vi "FPGA SPI_Configure.vi"(8 "error in":errorcluster, 9 "Configuration Cluster":T2={"CS"=1, "Clock Rate (Hz)"=50000.0, "Clock Mode"=0, "CS Active State"=FALSE} {"CS" items=["0"=1, "1"=2, "2"=4, "3"=8, "4"=16, "5"=32, "6"=64, "7"=128]; "Clock Mode" items=["0", "1", "2", "3"]}, 10 "Port":u8, 11 "FPGA VI Reference":T1) -> (0 "error out":errorcluster, 2 "Actual Rate (Hz)":dbl, 3 "FPGA VI Reference Out":T1)   [LabVIEW 2011]
uses:
  <vilib>/rvi/interface/nirviReadWriteControl/nirviReadWriteControl.xnode
  FPGA/Controls/FPGA SPI_Cmd.ctl
  Controls/FPGA SPI_FPGA Ref.ctl
  Controls/FPGA SPI_SPI Configuration Cluster.ctl
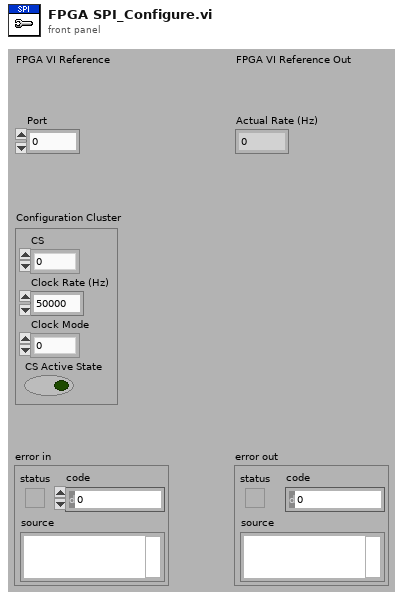
[diagram p1: front panel]
types:
  T1 = typedef "FPGA SPI_FPGA Ref.ctl" = refnum<k20>
  T2 = typedef "FPGA SPI_SPI Configuration Cluster.ctl" = cluster{"CS":u8, "Clock Rate (Hz)":dbl, "Clock Mode":u8, "CS Active State":bool}
  T3 = typedef "FPGA SPI_Cmd.ctl" = enum8{"Idle", "Write/Read SPI", "Configure"}
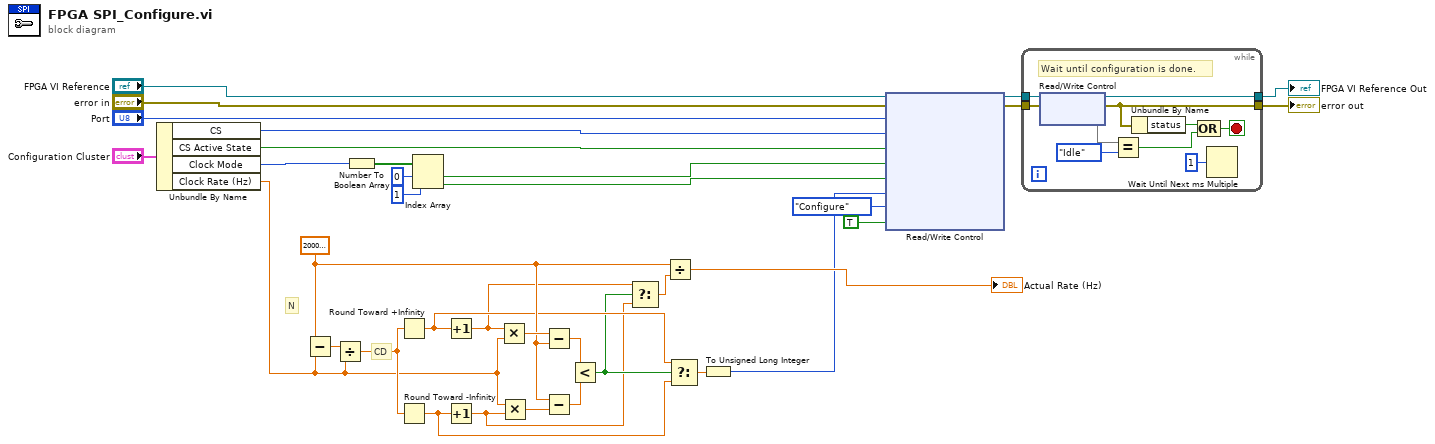
[diagram p0: block diagram]
diagram:
  w26 = 20000000.0 ("10M")
  # "CD"
  # "N"
  n1 = Unbundle By Name("Configuration Cluster") -> ("CS"=w31:u8, "CS Active State"=w8:bool, "Clock Mode"=w9:u8, "Clock Rate (Hz)"=w15:dbl)
  n2 = Subtract(x=w26, y=w15) -> (x-y=w25:dbl)
  n3 = Divide(x=w25, y=w15) -> (x/y=w24:dbl)
  n4 = Number To Boolean Array(number=w9) -> (Boolean array=w14:bool[])
  n5 = Round Toward +Infinity(x=w24) -> (ceil(x): smallest int >= x=w23:dbl)
  n6 = Round Toward -Infinity(1:w24) -> (0:w22:dbl)
  n7 = Index Array(array=w14, index #1=0 ("index"), index #2=1 ("index")) -> (element #1=w11:bool, element #2=w10:bool)
  n8 = Increment(x=w23) -> (x+1=w18:dbl)
  n9 = Increment(x=w22) -> (x+1=w19:dbl)
  n10 = Multiply(x=w18, y=w15) -> (x*y=w30:dbl)
  n11 = Multiply(x=w15, y=w19) -> (x*y=w29:dbl)
  n12 = Subtract(x=w30, y=w26) -> (x-y=w27:dbl)
  n13 = Subtract(x=w26, y=w29) -> (x-y=w28:dbl)
  n14 = Less?(x=w27, y=w28) -> (x < y?=w20:bool)
  n15 = Select(t=w18, s=w20, f=w19) -> (s? t:f=w21:dbl)
  n16 = Divide(x=w26, y=w21) -> (x/y=→"Actual Rate (Hz)":dbl)
  n17 = Select(t=w23, s=w20, f=w22) -> (s? t:f=w16:dbl)
  n18 = To Unsigned Long Integer(number=w16) -> (unsigned 32bit integer=w7:u32)
  n19 = xnode "Read/Write Control"("FPGA VI Reference In"="FPGA VI Reference", "error in"="error in", "SPI_Port"="Port", "SPI_CS"=w31, "SPI_CS Active State"=w8, "SPI_CPHA"=w11, "SPI_CPOL"=w10, "SPI_Clock Divider"=w7, "SPI_Cmd"=FPGA_SPI_Cmd."Configure" ("Cmd"), "SPI_Start"=TRUE ("Start")) -> ("FPGA VI Reference Out"=w4:T1, "error out"=w2:errorcluster)
  n20 = while {
    tunnel: w4 -> [w45]
    tunnel: [w44] -> w3
    tunnel: w2 -> [w43]
    tunnel: [w40] -> w1
    stop <- w37 stop-if-true
    # "Wait until configuration is done."
    n21 = xnode "Read/Write Control"("FPGA VI Reference In"=w45, "error in"=w43) -> ("FPGA VI Reference Out"=w44:T1, "error out"=w40:errorcluster, "SPI_Cmd"=w42)
    n22 = Equal?(x=w42, y=FPGA_SPI_Cmd."Idle") -> (x = y?=w38:bool)
    n23 = Unbundle By Name(w40) -> ("status"=w39:bool)
    n24 = Compound Arithmetic op=OR(w39, w38) -> (w37:bool)
    n25 = Wait Until Next ms Multiple(millisecond multiple=u32 1) -> ()  [unwired: 1 out]
  }
  "error out" <- w1
  "FPGA VI Reference Out" <- w3
